vi "dsdll_check_instance.vi"(8 "error in":errorcluster, 11 "dsdll instance in":T1) -> (0 "error out":errorcluster, 2 "empty instance handle":bool, 3 "dsdll instance out":T1)   [LabVIEW 2020, in "dsdll.lvlib"]
doc: "Checks is DSDLL instance was already initialized."
uses:
  dsdll.lvlib
  dsdll_instance.ctl
  dsdll_device_record.ctl
  <vilib>/Utility/error.llb/Error Cluster From Error Code.vi
  <vilib>/ErrorRing/Error Ring.xnode
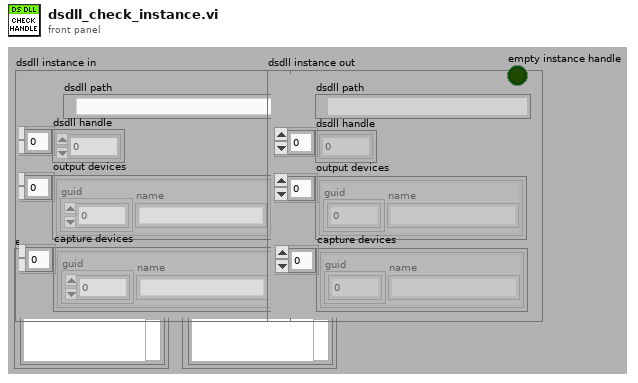
[diagram p1: front panel]
types:
  T1 = typedef "dsdll.lvlib/dsdll_instance.ctl" = cluster{"dsdll path":path, "dsdll handle":u8[], "output devices":T2[], "capture devices":T2[]}
  T2 = typedef "dsdll.lvlib/dsdll_device_record.ctl" = cluster{"guid":u8[], "name":string}
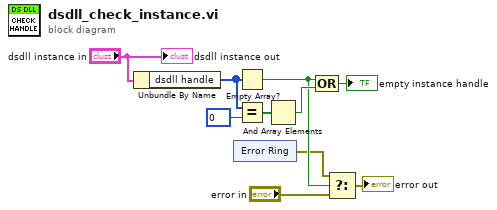
[diagram p0: block diagram]
diagram:
  n1 = Unbundle By Name("dsdll instance in") -> ("dsdll handle"=w9:u8[])
  n2 = xnode "Error Ring"() -> ("error out"=w2:errorcluster)
  n3 = Empty Array?(array=w9) -> (empty?=w3:bool)
  n4 = Equal?(x=w9, y=u8 0) -> (x = y?=w8:bool[])
  n5 = And Array Elements(Boolean array=w8) -> (logical AND=w7:bool)
  n6 = Compound Arithmetic op=OR(w3, w7) -> (→"empty instance handle":bool)
  n7 = Select(t=w2, s=w3, f="error in") -> (s? t:f=→"error out":errorcluster)
  "dsdll instance out" <- "dsdll instance in"
